vi "GetProjectConditionalDeactivationValues.vi"(8 "Fehler (Eingang, kein Fehler)":errorcluster, 11 "Projekt Referenz":refnum<vi>) -> (0 "Fehler (Ausgang)":errorcluster, 1 "Values aus Projekt":string[](array[string]), 2 "Keys aus Projekt":string[](array[string]), 3 "Projekt Referenz":refnum<vi>, 4 "Daten":string)   [LabVIEW 2020, in "ConditionalDeactivation.lvlib"]
uses:
  ConditionalDeactivation.lvlib
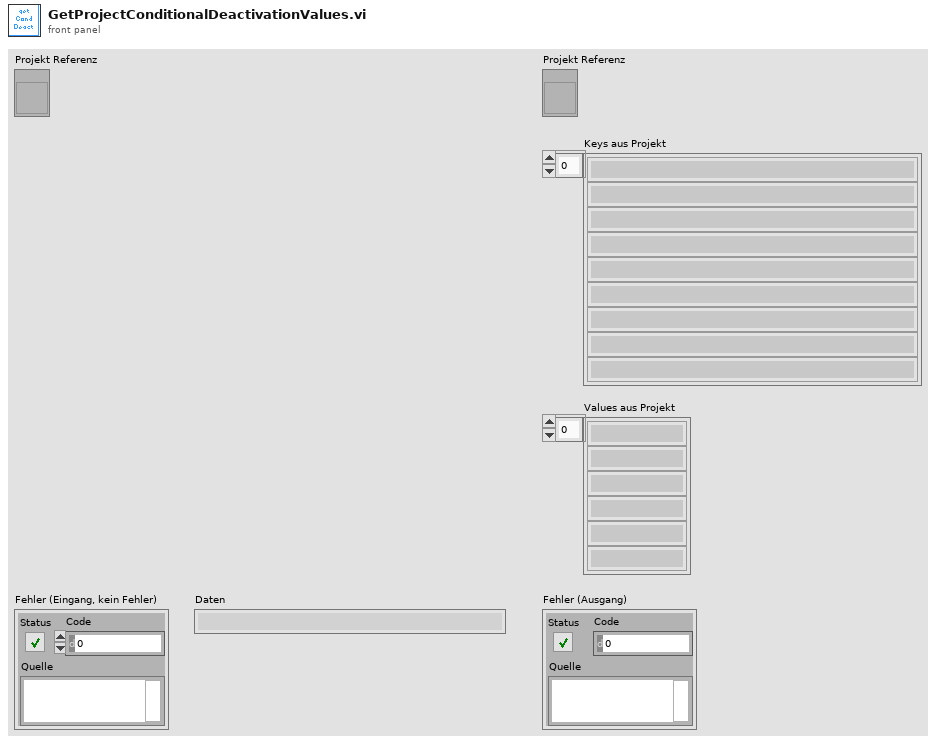
[diagram p1: front panel]
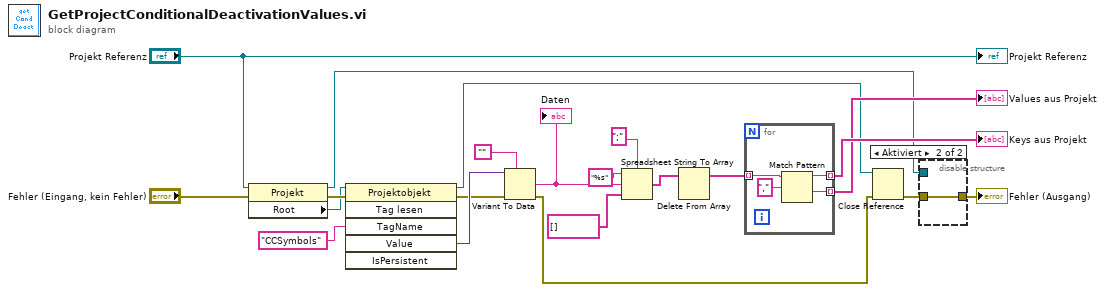
[diagram p0: block diagram]
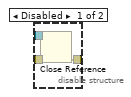
[diagram p2: hidden frame]
diagram:
  n1 = property class="Projekt"(reference="Projekt Referenz", error in="Fehler (Eingang, kein Fehler)") -> (reference out=w3:refnum<vi>, error out=w19:errorcluster, "Root"=w15:refnum<vi>)
  n2 = invoke class="Projektobjekt" method="Tag lesen"(reference=w15, error in=w19, "TagName"="CCSymbols" ("Tag-Name")) -> (reference out=w1:refnum<vi>, error out=w16:errorcluster, "Value"=w18:variant)  [unwired: 3 in, 3 out]
  n3 = Variant To Data(error in=w16, type="", Variant=w18) -> (data=w9:string, error out=w2:errorcluster)
  "Daten" <- w9
  n4 = Spreadsheet String To Array(delimiter (Tab)=";" ("Regulärer Ausdruck"), format string="%s" ("Format-String"), spreadsheet string=w9, array type (2D Dbl)=string[] []) -> (array=w8:string[])
  n5 = Delete From Array(array=w8) -> (array with subset deleted=w7:string[])  [unwired: 2 in, 1 out]
  n6 = for {
    tunnel: w7 -> [w25] mode=indexing
    tunnel: [w23] -> w6 mode=indexing
    tunnel: [w22] -> w5 mode=indexing
    n7 = Match Pattern(string=w25, regular expression="," ("Regulärer Ausdruck")) -> (before substring=w23:string, after substring=w22:string)  [unwired: 1 in, 2 out]
  }
  "Keys aus Projekt" <- w6
  "Values aus Projekt" <- w5
  n8 = Close Reference(reference=w1, error in (no error)=w2) -> (error out=w14:errorcluster)
  n9 = disable-structure shown="Aktiviert" {
    disable-tunnel: w14 -> [w28 w29]
    disable-tunnel: [w27 w29] -> w13
    disable-tunnel: w3 -> [w26 _]
    frame Disabled {
      n10 = Close Reference(reference=w26, error in (no error)=w28) -> (error out=w27:errorcluster)
    }
    frame Enabled {
    }
  }
  "Fehler (Ausgang)" <- w13
  "Projekt Referenz" <- "Projekt Referenz"
